vi "GET_3rd party Templates.vi"(8 "error in (no error)":errorcluster {"code" min=0 max=0}, 11 "Settings.lvclass in":refnum<class "Settings.lvclass">) -> (0 "error out":errorcluster {"code" min=0 max=0}, 2 "3rd party Templates":T1, 3 "Settings.lvclass out":refnum<class "Settings.lvclass">)   [LabVIEW 2021, in "Settings.lvclass"]
uses:
  <resource>/plugins/NIIconEditor/Class/Settings/Settings.lvclass
  <resource>/plugins/NIIconEditor/Class/Settings/Settings.lvclass/Settings.ctl
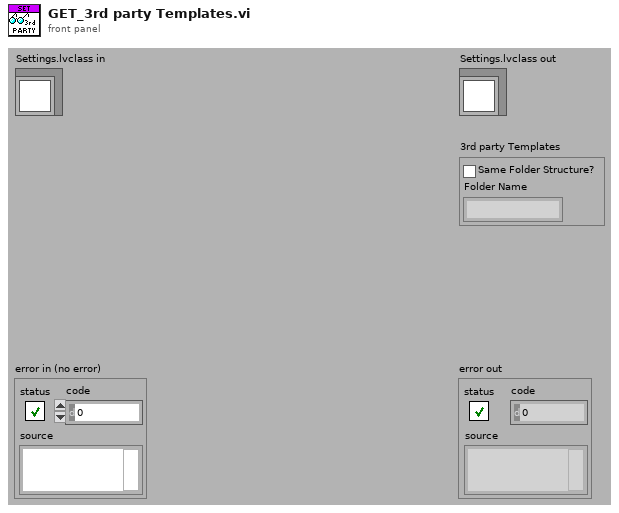
[diagram p1: front panel]
types:
  T1 = cluster{"Same Folder Structure?":bool, "Folder Name":string}
  T2 = cluster{"Store 3rd party Templates?":bool, "Folder Name":string}
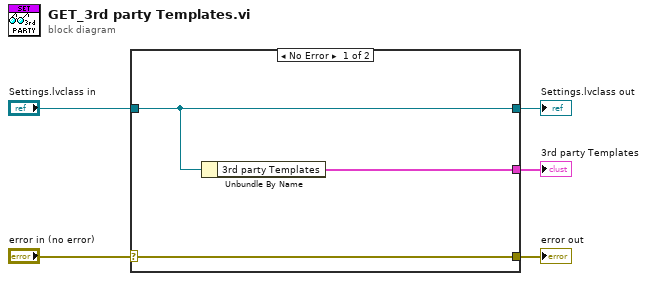
[diagram p0: block diagram]
diagram:
  n1 = case shown="No Error" "error in (no error)" {
    selector: "error in (no error)" -> [w8 w9]
    tunnel: [w8 w9] -> w4
    tunnel: [w7 w10] -> w2
    tunnel: "Settings.lvclass in" -> [w7 w10]
    tunnel: [w6 _] -> w1
    frame No Error {
      n2 = Unbundle By Name(w7) -> ("3rd party Templates"=w6:T2)
    }
    frame Error {
    }
  }
  "error out" <- w4
  "Settings.lvclass out" <- w2
  "3rd party Templates" <- w1
